vi "Configure Multi Eval Meas Limit FERR.vi"(6 "Limit Value (0.1)":dbl=0.1 format="%^.3e", 7 "Limit Check Enabled (Value)":i32(ring)=2 items=["Off", "On", "Value"], 8 "error in (no error)":errorcluster, 9 "Modulation (Pi/2-BPSK)":i32(ring) items=["Pi/2-BPSK", "Pi/2-BPSK With Shaping", "QPSK", "16-QAM", "64-QAM", "256-QAM"], 10 "Instance (1)":T1=1, 11 "VISA resource name":refnum<visa-resource-name>) -> (0 "error out":errorcluster, 3 "VISA resource name out":refnum<visa-resource-name>)   [LabVIEW 2020, in "Rohde&Schwarz CMWXP NR FR1 Measurement.lvlib"]
doc: "Defines an upper limit for the carrier frequency error.\n\nAttributes:\nRSCMWXPNRFR1M_ATTR_MULTI_EVAL_MEAS_LIMIT_PI_2_FERR\nRSCMWXPNRFR1M_ATTR_MULTI_EVAL_MEAS_LIMIT_PI_2_FERR_ENABLED\nRSCMWXPNRFR1M_ATTR_MULTI_EVAL_MEAS_LIMIT_BPSK_SHAPING_FERR\nRSCMWXPNRFR1M_ATTR_MULTI_EVAL_MEAS_LIMIT_BPSK_SHAPING_FERR_ENABLED\nRSCMWXPNRFR1M_ATTR_MULTI_EVAL_MEAS_LIMIT_QPSK_FERR\nRSCMWXPNRFR1M_ATTR_MULTI_EVAL_MEAS_LIMIT_QPSK_FERR_ENABLED\nRSCMWXPNRFR1M_ATTR_MULTI_EVAL_MEAS_LIMIT_QAM_FERR\nRSCMWXPNRFR1M_ATTR_MULTI_EVAL_MEAS_LIMIT_QAM_FERR_ENABLED\n\nRemote-control commands:\nCONFigure:NRSub:MEAS<i>:MEValuation:LIMit:PHBPsk:FERRor\nCONFigure:NRSub:MEAS<i>:MEValuation:LIMit:BPWShaping:FERRor\nCONFigure:NRSub:MEAS<i>:MEValuation:LIMit:QPSK:FERRor\nCONFigure:NRSub:MEAS<i>:MEValuation:LIMit:QAM<order>:FERRor"
uses:
  <instrlib>/Rohde&Schwarz CMWXP NR FR1 Measurement/Rohde&Schwarz CMWXP NR FR1 Measurement.lvlib
  <instrlib>/Rohde&Schwarz CMWXP NR FR1 Measurement/Private/_Instance.ctl
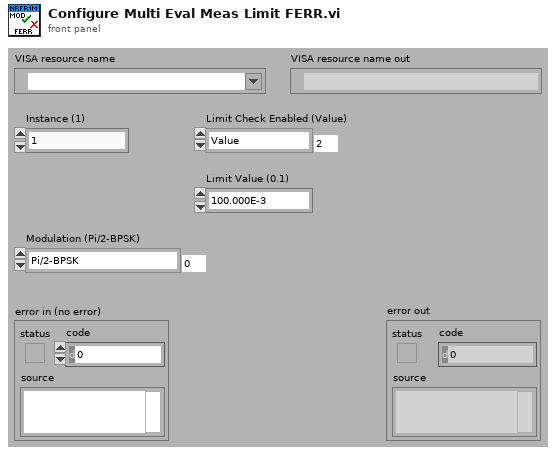
[diagram p1: front panel]
types:
  T1 = typedef "Rohde&Schwarz CMWXP NR FR1 Measurement.lvlib/_Instance.ctl" = i32
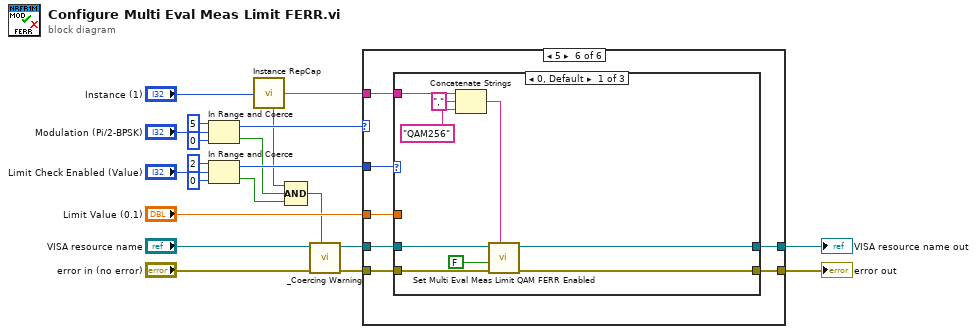
[diagram p0: block diagram]
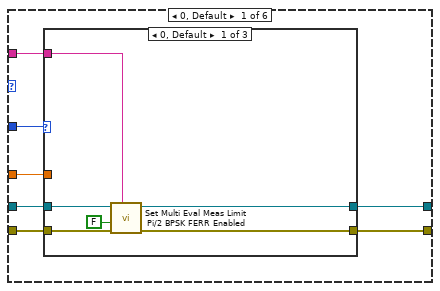
[diagram p2: hidden frame]
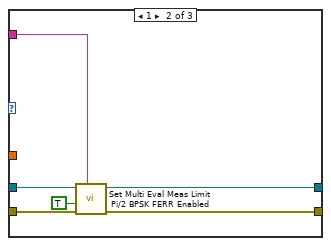
[diagram p3: hidden frame]
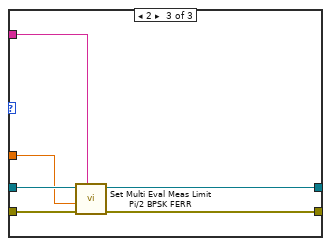
[diagram p4: hidden frame]
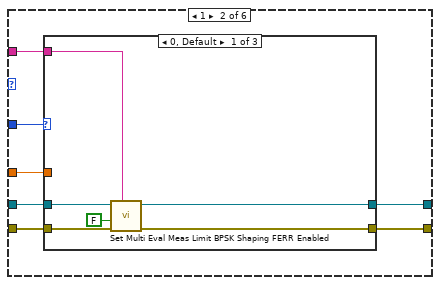
[diagram p5: hidden frame]
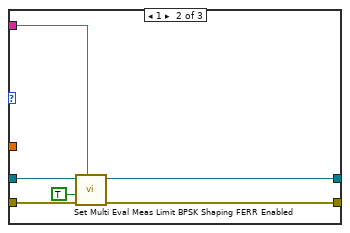
[diagram p6: hidden frame]
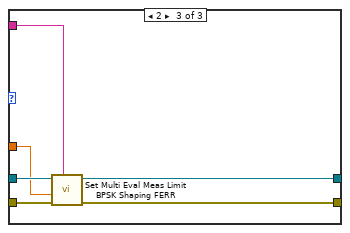
[diagram p7: hidden frame]
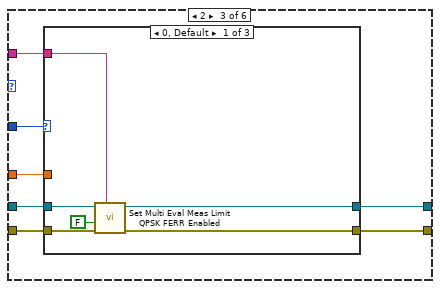
[diagram p8: hidden frame]
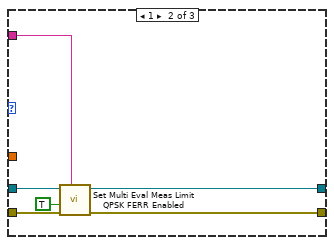
[diagram p9: hidden frame]
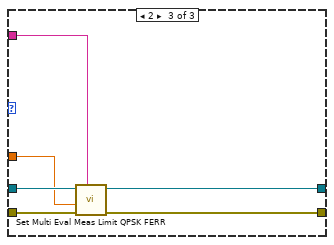
[diagram p10: hidden frame]
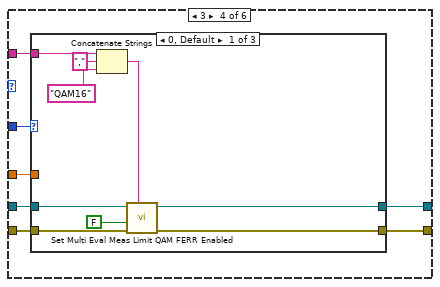
[diagram p11: hidden frame]
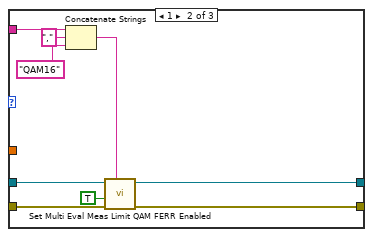
[diagram p12: hidden frame]
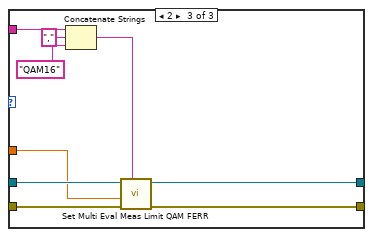
[diagram p13: hidden frame]
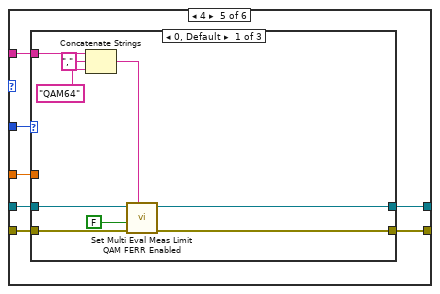
[diagram p14: hidden frame]
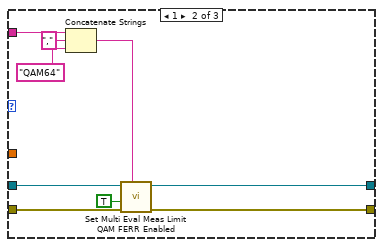
[diagram p15: hidden frame]
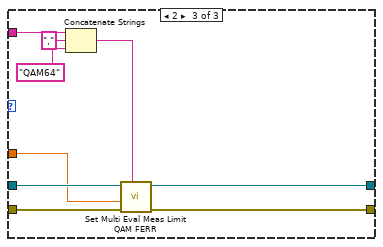
[diagram p16: hidden frame]
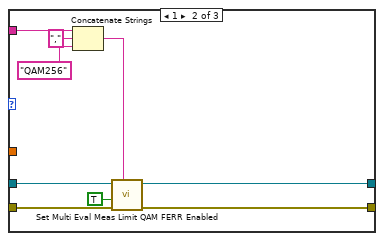
[diagram p17: hidden frame]
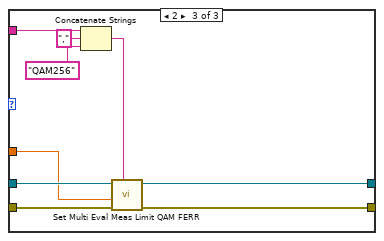
[diagram p18: hidden frame]
diagram:
  n1 = In Range and Coerce(upper limit=5, x="Modulation (Pi/2-BPSK)", lower limit=0) -> (coerced(x)=w10:i32, In Range?=w2:bool)
  n2 = In Range and Coerce(upper limit=2, x="Limit Check Enabled (Value)", lower limit=0) -> (coerced(x)=w9:i32, In Range?=w3:bool)
  n3 = call <instrlib>:"Instance RepCap.vi"("Instance In"="Instance (1)") -> ("In Range?"=w1:bool, "RepCap Identifier Out"=w20:string)  [unwired: 1 in]
  n4 = Compound Arithmetic op=AND(w1, w2, w3) -> (w4:bool)
  n5 = call <instrlib>:"_Coercing Warning.vi"("In Range?"=w4, "error in (no error)"="error in (no error)", "VISA resource name"="VISA resource name") -> ("error out"=w14:errorcluster, "VISA resource name out"=w13:refnum<visa-resource-name>)  [unwired: 7 in]
  n6 = case shown="5" w10 {
    tunnel: [w22 w47 w72 w97 w131 w165] -> w17
    tunnel: [w23 w48 w73 w98 w132 w166] -> w18
    tunnel: w20 -> [w26 w51 w76 w101 w135 w169]
    tunnel: w9 -> [w28 w53 w78 w103 w137 w171]
    tunnel: w13 -> [w27 w52 w77 w102 w136 w170]
    tunnel: w14 -> [w25 w50 w75 w100 w134 w168]
    tunnel: "Limit Value (0.1)" -> [w24 w49 w74 w99 w133 w167]
    frame 0, Default {
      n7 = case shown="0, Default" w28 {
        tunnel: w27 -> [w32 w38 w44]
        tunnel: [w29 w35 w41] -> w22
        tunnel: [w30 w36 w42] -> w23
        tunnel: w26 -> [w34 w40 w46]
        tunnel: w25 -> [w33 w39 w45]
        tunnel: w24 -> [_ _ w43]
        frame 0, Default {
          n8 = call "Set Multi Eval Meas Limit Pi/2 BPSK FERR Enabled"("Repeated Capabilities"=w34, "error in (no error)"=w33, "Multi Eval Meas Limit Pi/2 BPSK FERR Enabled (OFF)"=FALSE, "instrument handle"=w32) -> ("error out"=w29:errorcluster, "instrument handle out"=w30:refnum<visa-resource-name>)  [unwired: 6 in]
        }
        frame 1 {
          n9 = call "Set Multi Eval Meas Limit Pi/2 BPSK FERR Enabled"("Repeated Capabilities"=w40, "error in (no error)"=w39, "Multi Eval Meas Limit Pi/2 BPSK FERR Enabled (OFF)"=TRUE, "instrument handle"=w38) -> ("error out"=w35:errorcluster, "instrument handle out"=w36:refnum<visa-resource-name>)  [unwired: 6 in]
        }
        frame 2 {
          n10 = call "Set Multi Eval Meas Limit Pi/2 BPSK FERR"("Repeated Capabilities"=w46, "error in (no error)"=w45, "Multi Eval Meas Limit Pi/2 BPSK FERR (0.0)"=w43, "instrument handle"=w44) -> ("error out"=w41:errorcluster, "instrument handle out"=w42:refnum<visa-resource-name>)  [unwired: 6 in]
        }
      }
    }
    frame 1 {
      n11 = case shown="0, Default" w53 {
        tunnel: w52 -> [w57 w63 w69]
        tunnel: [w54 w60 w66] -> w47
        tunnel: [w55 w61 w67] -> w48
        tunnel: w51 -> [w59 w65 w71]
        tunnel: w50 -> [w58 w64 w70]
        tunnel: w49 -> [_ _ w68]
        frame 0, Default {
          n12 = call "Set Multi Eval Meas Limit BPSK Shaping FERR Enabled"("Repeated Capabilities"=w59, "error in (no error)"=w58, "Multi Eval Meas Limit BPSK Shaping FERR Enabled (OFF)"=FALSE ("Multi Eval Meas Limit Pi/2 BPSK FERR Enabled (OFF)"), "instrument handle"=w57) -> ("error out"=w54:errorcluster, "instrument handle out"=w55:refnum<visa-resource-name>)  [unwired: 6 in]
        }
        frame 1 {
          n13 = call "Set Multi Eval Meas Limit BPSK Shaping FERR Enabled"("Repeated Capabilities"=w65, "error in (no error)"=w64, "Multi Eval Meas Limit BPSK Shaping FERR Enabled (OFF)"=TRUE ("Multi Eval Meas Limit Pi/2 BPSK FERR Enabled (OFF)"), "instrument handle"=w63) -> ("error out"=w60:errorcluster, "instrument handle out"=w61:refnum<visa-resource-name>)  [unwired: 6 in]
        }
        frame 2 {
          n14 = call "Set Multi Eval Meas Limit BPSK Shaping FERR"("Repeated Capabilities"=w71, "error in (no error)"=w70, "Multi Eval Meas Limit BPSK Shaping FERR (0.0)"=w68, "instrument handle"=w69) -> ("error out"=w66:errorcluster, "instrument handle out"=w67:refnum<visa-resource-name>)  [unwired: 6 in]
        }
      }
    }
    frame 2 {
      n15 = case shown="0, Default" w78 {
        tunnel: w77 -> [w82 w88 w94]
        tunnel: [w79 w85 w91] -> w72
        tunnel: [w80 w86 w92] -> w73
        tunnel: w76 -> [w84 w90 w96]
        tunnel: w75 -> [w83 w89 w95]
        tunnel: w74 -> [_ _ w93]
        frame 0, Default {
          n16 = call "Set Multi Eval Meas Limit QPSK FERR Enabled"("Repeated Capabilities"=w84, "error in (no error)"=w83, "Multi Eval Meas Limit QPSK FERR Enabled (OFF)"=FALSE ("Multi Eval Meas Limit Pi/2 BPSK FERR Enabled (OFF)"), "instrument handle"=w82) -> ("error out"=w79:errorcluster, "instrument handle out"=w80:refnum<visa-resource-name>)  [unwired: 6 in]
        }
        frame 1 {
          n17 = call "Set Multi Eval Meas Limit QPSK FERR Enabled"("Repeated Capabilities"=w90, "error in (no error)"=w89, "Multi Eval Meas Limit QPSK FERR Enabled (OFF)"=TRUE ("Multi Eval Meas Limit Pi/2 BPSK FERR Enabled (OFF)"), "instrument handle"=w88) -> ("error out"=w85:errorcluster, "instrument handle out"=w86:refnum<visa-resource-name>)  [unwired: 6 in]
        }
        frame 2 {
          n18 = call "Set Multi Eval Meas Limit QPSK FERR"("Repeated Capabilities"=w96, "error in (no error)"=w95, "Multi Eval Meas Limit QPSK FERR (0.0)"=w93, "instrument handle"=w94) -> ("error out"=w91:errorcluster, "instrument handle out"=w92:refnum<visa-resource-name>)  [unwired: 6 in]
        }
      }
    }
    frame 3 {
      n19 = case shown="0, Default" w103 {
        tunnel: w102 -> [w111 w120 w129]
        tunnel: [w108 w117 w126] -> w97
        tunnel: [w109 w118 w127] -> w98
        tunnel: w101 -> [w107 w114 w123]
        tunnel: w100 -> [w112 w121 w130]
        tunnel: w99 -> [_ _ w128]
        frame 0, Default {
          n20 = Concatenate Strings(w107, "," ("string"), "QAM16" ("string")) -> (w104:string)
          n21 = call "Set Multi Eval Meas Limit QAM FERR Enabled"("Repeated Capabilities"=w104, "error in (no error)"=w112, "Multi Eval Meas Limit QAM FERR Enabled (OFF)"=FALSE ("Multi Eval Meas Limit Pi/2 BPSK FERR Enabled (OFF)"), "instrument handle"=w111) -> ("error out"=w108:errorcluster, "instrument handle out"=w109:refnum<visa-resource-name>)  [unwired: 6 in]
        }
        frame 1 {
          n22 = Concatenate Strings(w114, "," ("string"), "QAM16" ("string")) -> (w113:string)
          n23 = call "Set Multi Eval Meas Limit QAM FERR Enabled"("Repeated Capabilities"=w113, "error in (no error)"=w121, "Multi Eval Meas Limit QAM FERR Enabled (OFF)"=TRUE ("Multi Eval Meas Limit Pi/2 BPSK FERR Enabled (OFF)"), "instrument handle"=w120) -> ("error out"=w117:errorcluster, "instrument handle out"=w118:refnum<visa-resource-name>)  [unwired: 6 in]
        }
        frame 2 {
          n24 = Concatenate Strings(w123, "," ("string"), "QAM16" ("string")) -> (w122:string)
          n25 = call "Set Multi Eval Meas Limit QAM FERR"("Repeated Capabilities"=w122, "error in (no error)"=w130, "Multi Eval Meas Limit QAM FERR (0.0)"=w128, "instrument handle"=w129) -> ("error out"=w126:errorcluster, "instrument handle out"=w127:refnum<visa-resource-name>)  [unwired: 6 in]
        }
      }
    }
    frame 4 {
      n26 = case shown="0, Default" w137 {
        tunnel: w136 -> [w145 w154 w163]
        tunnel: [w142 w151 w160] -> w131
        tunnel: [w143 w152 w161] -> w132
        tunnel: w135 -> [w141 w148 w157]
        tunnel: w134 -> [w146 w155 w164]
        tunnel: w133 -> [_ _ w162]
        frame 0, Default {
          n27 = Concatenate Strings(w141, "," ("string"), "QAM64" ("string")) -> (w138:string)
          n28 = call "Set Multi Eval Meas Limit QAM FERR Enabled"("Repeated Capabilities"=w138, "error in (no error)"=w146, "Multi Eval Meas Limit QAM FERR Enabled (OFF)"=FALSE ("Multi Eval Meas Limit Pi/2 BPSK FERR Enabled (OFF)"), "instrument handle"=w145) -> ("error out"=w142:errorcluster, "instrument handle out"=w143:refnum<visa-resource-name>)  [unwired: 6 in]
        }
        frame 1 {
          n29 = Concatenate Strings(w148, "," ("string"), "QAM64" ("string")) -> (w147:string)
          n30 = call "Set Multi Eval Meas Limit QAM FERR Enabled"("Repeated Capabilities"=w147, "error in (no error)"=w155, "Multi Eval Meas Limit QAM FERR Enabled (OFF)"=TRUE ("Multi Eval Meas Limit Pi/2 BPSK FERR Enabled (OFF)"), "instrument handle"=w154) -> ("error out"=w151:errorcluster, "instrument handle out"=w152:refnum<visa-resource-name>)  [unwired: 6 in]
        }
        frame 2 {
          n31 = Concatenate Strings(w157, "," ("string"), "QAM64" ("string")) -> (w156:string)
          n32 = call "Set Multi Eval Meas Limit QAM FERR"("Repeated Capabilities"=w156, "error in (no error)"=w164, "Multi Eval Meas Limit QAM FERR (0.0)"=w162, "instrument handle"=w163) -> ("error out"=w160:errorcluster, "instrument handle out"=w161:refnum<visa-resource-name>)  [unwired: 6 in]
        }
      }
    }
    frame 5 {
      n33 = case shown="0, Default" w171 {
        tunnel: w170 -> [w179 w188 w197]
        tunnel: [w176 w185 w194] -> w165
        tunnel: [w177 w186 w195] -> w166
        tunnel: w169 -> [w175 w182 w191]
        tunnel: w168 -> [w180 w189 w198]
        tunnel: w167 -> [_ _ w196]
        frame 0, Default {
          n34 = Concatenate Strings(w175, "," ("string"), "QAM256" ("string")) -> (w172:string)
          n35 = call "Set Multi Eval Meas Limit QAM FERR Enabled"("Repeated Capabilities"=w172, "error in (no error)"=w180, "Multi Eval Meas Limit QAM FERR Enabled (OFF)"=FALSE ("Multi Eval Meas Limit Pi/2 BPSK FERR Enabled (OFF)"), "instrument handle"=w179) -> ("error out"=w176:errorcluster, "instrument handle out"=w177:refnum<visa-resource-name>)  [unwired: 6 in]
        }
        frame 1 {
          n36 = Concatenate Strings(w182, "," ("string"), "QAM256" ("string")) -> (w181:string)
          n37 = call "Set Multi Eval Meas Limit QAM FERR Enabled"("Repeated Capabilities"=w181, "error in (no error)"=w189, "Multi Eval Meas Limit QAM FERR Enabled (OFF)"=TRUE ("Multi Eval Meas Limit Pi/2 BPSK FERR Enabled (OFF)"), "instrument handle"=w188) -> ("error out"=w185:errorcluster, "instrument handle out"=w186:refnum<visa-resource-name>)  [unwired: 6 in]
        }
        frame 2 {
          n38 = Concatenate Strings(w191, "," ("string"), "QAM256" ("string")) -> (w190:string)
          n39 = call "Set Multi Eval Meas Limit QAM FERR"("Repeated Capabilities"=w190, "error in (no error)"=w198, "Multi Eval Meas Limit QAM FERR (0.0)"=w196, "instrument handle"=w197) -> ("error out"=w194:errorcluster, "instrument handle out"=w195:refnum<visa-resource-name>)  [unwired: 6 in]
        }
      }
    }
  }
  "error out" <- w17
  "VISA resource name out" <- w18
